vi "OAT Calc dM.vi"(7 "recieved":i32, 8 "oversampling rate":enum8{"2", "4", "8", "16"}(ring)=enum."4", 9 "window length":i32=2048 min=2, 11 "signal length":i32) -> (0 "dM":i32, 1 "actual window length":i32, 3 "# of Gabor windows":i32, 5 "left":i32)   [LabVIEW 2017]
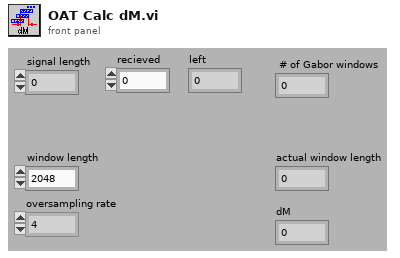
[diagram p1: front panel]
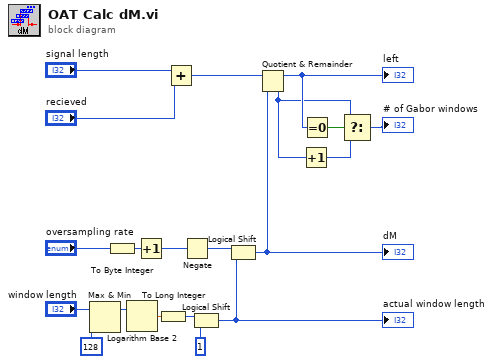
[diagram p0: block diagram]
diagram:
  n1 = Max & Min(x="window length", y=128) -> (max(x,y)=w12:i32)  [unwired: 1 out]
  n2 = To Byte Integer(number="oversampling rate") -> (8bit integer=w19:i8)
  n3 = Logarithm Base 2(1:w12) -> (0:w16:dbl)
  n4 = Increment(x=w19) -> (x+1=w10:i8)
  n5 = To Long Integer(number=w16) -> (32bit integer=w15:i32)
  n6 = Add(x="signal length", y="recieved") -> (x+y=w6:i32)
  n7 = Negate(x=w10) -> (-x=w18:i8)
  n8 = Logical Shift(y=w15, x=1) -> (x << y=w13:i32)
  "actual window length" <- w13
  n9 = Logical Shift(y=w18, x=w13) -> (x << y=w7:i32)
  "dM" <- w7
  n10 = Quotient & Remainder(x=w6, y=w7) -> (x-y*floor(x/y)=w5:i32, floor(x/y)=w3:i32)
  "left" <- w5
  n11 = Increment(x=w3) -> (x+1=w2:i32)
  n12 = Equal To 0?(x=w5) -> (x = 0?=w4:bool)
  n13 = Select(t=w3, s=w4, f=w2) -> (s? t:f=→"# of Gabor windows":i32)
